vi "loadandrun_subvi.vi"(0 "path":path caption="路径", 1 "run?":bool caption="运行？", 3 "error in (no error)":errorcluster caption="错误输入（无错误）") -> (7 "vi refnum out":refnum<vi> caption="VI引用句柄输出", 10 "error out":errorcluster caption="错误输出")   [LabVIEW 2012]
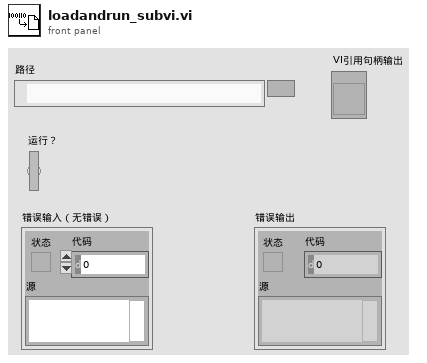
[diagram p1: front panel]
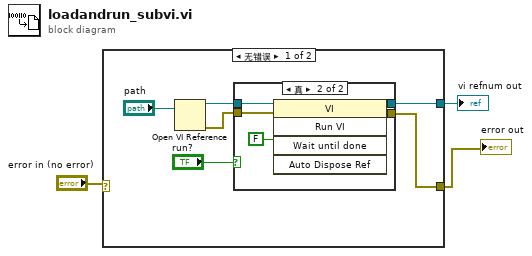
[diagram p0: block diagram]
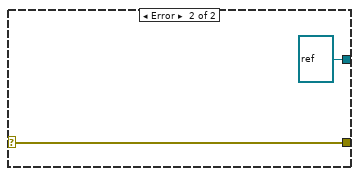
[diagram p3: hidden frame]
diagram:
  n1 = case shown="无错误" "error in (no error)" {
    selector: "error in (no error)" -> [_ w17]
    tunnel: [w6 refnum<vi> refnum] -> w2
    tunnel: [w4 w17] -> w1
    frame No Error {
      n2 = Open VI Reference(vi path="path") -> (vi reference=w7:refnum<vi>, error out=w5:errorcluster)  [unwired: 5 in]
      n3 = case shown="真" "run?" {
        tunnel: w7 -> [w11 w16]
        tunnel: [w11 w14] -> w6
        tunnel: w5 -> [w10 w13]
        tunnel: [w10 w12] -> w4
        frame False {
        }
        frame True {
          n4 = invoke class="VI" method="Run VI"(reference=w16, error in=w13, "Wait until done"=FALSE) -> (reference out=w14:refnum<vi>, error out=w12:errorcluster)  [unwired: 2 in, 3 out]
        }
      }
    }
    frame Error {
    }
  }
  "vi refnum out" <- w2
  "error out" <- w1
